vi "NI-XNET Frame&Log - Convert Single Frame (Raw to CAN).vi"(0 "converter  in":T3, 7 "raw frames":u8[](array[numeric]) format="%02x", 11 "error in":errorcluster) -> (4 "converter out":T3, 8 "CAN frame":T1 {"payload" format="%x"; "timestamp" format="%<%.7X\n%x>T"; "type" items=["CAN Data"=0, "CAN Remote"=1, "CAN Bus Error"=2, "Delay"=224, "Log Trigger"=225, "Start Trigger"=226]; "identifier" format="%x"}, 10 "valid?":bool, 15 "error out":errorcluster)   [LabVIEW 2014]
doc: "Convert array of raw frame data to a single CAN frame.\n\nIf no valid frame exists at the current index, the boolean \"valid?\" is false.\n\nUpon return, index is set to the start of the next CAN frame in raw data, or -1 if the end of the raw data was reached."
uses:
  NI-XNET Frame&Log - Converter.ctl
  <vilib>/xnet/xnet.llb/XNET Frame CAN.ctl
  <vilib>/xnet/xnet.llb/XNET Frame Type CAN.ctl
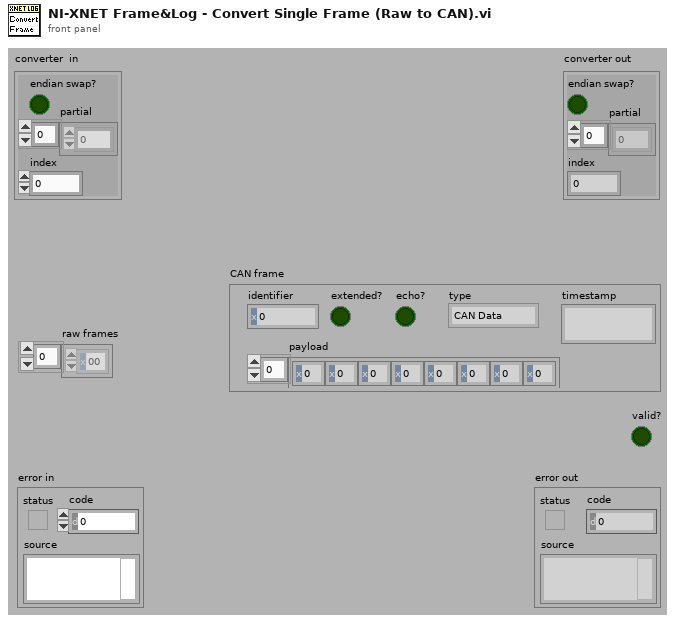
[diagram p1: front panel]
types:
  T1 = typedef "XNET Frame CAN.ctl" = cluster{"timestamp":timestamp, "payload":u8[], "identifier":u32, "type":T2, "extended?":bool, "echo?":bool}
  T2 = typedef "XNET Frame Type CAN.ctl" = u8
  T3 = typedef "NI-XNET Frame&Log - Converter.ctl" = cluster{"endian swap?":bool, "partial":u8[], "index":i32}
  T4 = enum16{"big-endian, network order", "native, host order", "little-endian"}
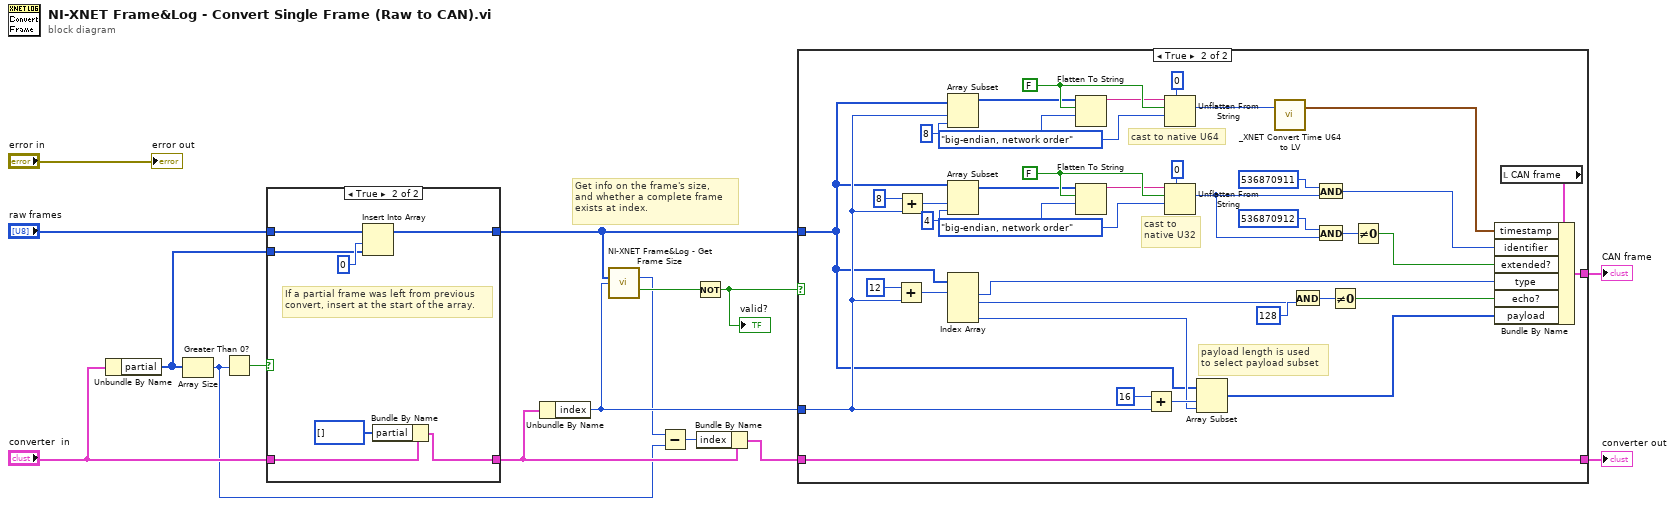
[diagram p0: block diagram]
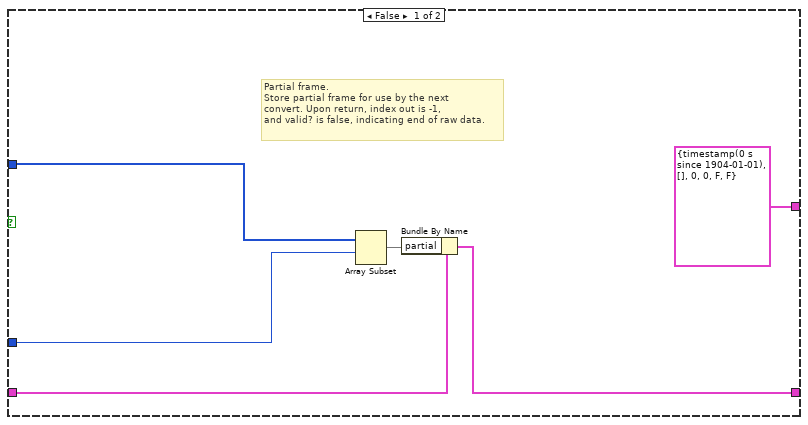
[diagram p3: hidden frame]
diagram:
  # "Get info on the frame's size,\nand whether a complete frame\nexists at index."
  n1 = Unbundle By Name("converter  in") -> ("partial"=w13:u8[])
  n2 = Array Size(array=w13) -> (size(s)=w1:i32)
  n3 = Greater Than 0?(x=w1) -> (x > 0?=w14:bool)
  n4 = case shown="True" w14 {
    tunnel: "converter  in" -> [w18 w24]
    tunnel: "raw frames" -> [w17 w20]
    tunnel: [w18 w23] -> w7
    tunnel: [w17 w19] -> w4
    tunnel: w13 -> [_ w21]
    frame False {
    }
    frame True {
      # "If a partial frame was left from previous\nconvert, insert at the start of the array."
      n5 = Insert Into Array(array=w20, index=0 ("index in"), new element=w21) -> (w19:u8[])
      n6 = Bundle By Name(cluster=w24, "partial"=u8[] []) -> (w23:T3)
    }
  }
  n7 = Unbundle By Name(w7) -> ("index"=w8:i32)
  n8 = call "NI-XNET Frame&Log - Get Frame Size.vi"("raw frames"=w4, "index"=w8) -> ("next index"=w2:i32, "partial?"=w11:bool)  [unwired: 12 out]
  n9 = Subtract(x=w2, y=w1) -> (x-y=w3:i32)
  n10 = Not(x=w11) -> (.not. x?=w10:bool)
  "valid?" <- w10
  n11 = Bundle By Name(cluster=w7, "index"=w3) -> (w6:T3)
  n12 = case shown="True" w10 {
    tunnel: w8 -> [w29 w40]
    tunnel: w4 -> [w30 w39]
    tunnel: [T1 {"timestamp"=timestamp(0 s since 1904-01-01), "payload"=[], "identifier"=0, "type"=0, "extended?"=FALSE, "echo?"=FALSE} ("CAN frame") w38] -> w15
    tunnel: w6 -> [w28 w69]
    tunnel: [w27 w69] -> w9
    frame False {
      # "Partial frame.\nStore partial frame for use by the next \nconvert. Upon return, index out is -1,\nand valid? is false, indicating end of raw data."
      n13 = Array Subset(array=w30, index=w29) -> (w31:u8[])  [unwired: 1 in]
      n14 = Bundle By Name(cluster=w28, "partial"=w31) -> (w27:T3)
    }
    frame True {
      w45 = T4."big-endian, network order" ("byte order (0:big-endian, network order)")
      w51 = T4."big-endian, network order" ("byte order (0:big-endian, network order)")
      w46 = FALSE ("prepend array or string size? (T)")
      w52 = FALSE ("prepend array or string size? (T)")
      # "payload length is used\nto select payload subset"
      # "cast to \nnative U32"
      # "cast to native U64"
      n15 = Add(x=12, y=w40) -> (x+y=w57:i32)
      n16 = Add(x=8, y=w40) -> (x+y=w59:i32)
      n17 = Array Subset(array=w39, index=w40, length=8) -> (w43:u8[])
      n18 = Array Subset(array=w39, index=w59, length=4) -> (w49:u8[])
      n19 = Index Array(array=w39, index #1=w57) -> (element #1=w56:u8, element #2=w33:u8, element #4=w53:u8)  [unwired: 3 in, 1 out]
      n20 = Flatten To String(anything=w43, prepend array or string size? (T)=w46, byte order (0:big-endian, network order)=w45) -> (data string=w44:string)  [unwired: 1 in, 2 out]
      n21 = Flatten To String(anything=w49, prepend array or string size? (T)=w52, byte order (0:big-endian, network order)=w51) -> (data string=w50:string)  [unwired: 1 in, 2 out]
      n22 = Add(x=16, y=w40) -> (x+y=w54:i32)
      n23 = Unflatten From String(type=u64 0 ("length"), binary string=w44, data includes array or string size? (T)=w46, byte order (0:big-endian, network order)=w45) -> (value=w41:u64)  [unwired: 1 in, 2 out]
      n24 = Unflatten From String(type=u32 0 ("length"), binary string=w50, data includes array or string size? (T)=w52, byte order (0:big-endian, network order)=w51) -> (value=w47:u32)  [unwired: 1 in, 2 out]
      n25 = Array Subset(array=w39, index=w54, length=w53) -> (w36:u8[])
      n26 = call <vilib>:"_XNET Convert Time U64 to LV.vi"("Time U64"=w41) -> ("Time LV"=w68:timestamp)  [unwired: 2 out]
      n27 = And(x=w33, y=u8 128) -> (x .and. y?=w35:u8)
      n28 = And(x=u32 536870911, y=w47) -> (x .and. y?=w65:u32)
      n29 = And(x=u32 536870912, y=w47) -> (x .and. y?=w64:u32)
      n30 = Not Equal To 0?(x=w35) -> (x != 0?=w32:bool)
      n31 = Not Equal To 0?(x=w64) -> (x != 0?=w63:bool)
      n32 = local read "CAN frame"() -> (w37:T1)
      n33 = Bundle By Name(cluster=w37, "timestamp"=w68, "identifier"=w65, "extended?"=w63, "type"=w56, "echo?"=w32, "payload"=w36) -> (w38:T1)
    }
  }
  "converter out" <- w9
  "CAN frame" <- w15
  "error out" <- "error in"
